vi "Moving_Statistic_Measurement.vi"(8 "error in (no error)":errorcluster, 10 "New_Measurement":dbl format="%#_13g", 11 "Moving_Mean in":refnum<class "Moving_Statistic.lvclass">) -> (0 "error out":errorcluster, 3 "Moving_Mean out":refnum<class "Moving_Statistic.lvclass">)   [LabVIEW 2021, in "Moving_Statistic.lvclass"]
uses:
  Moving_Statistic.lvclass
  Moving_Statistic.lvclass/Moving_Statistic.ctl
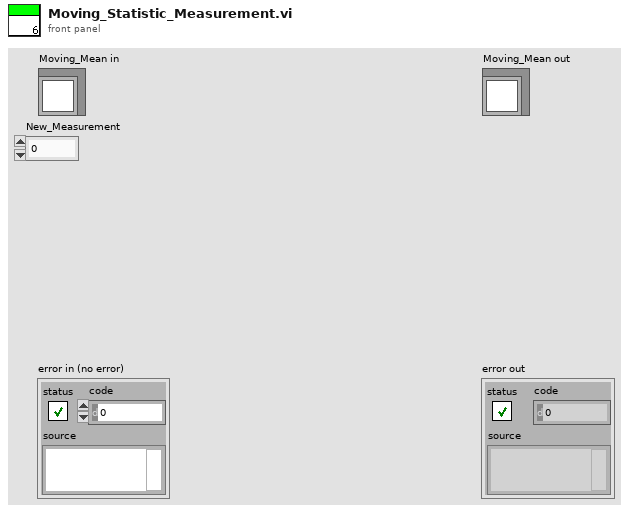
[diagram p1: front panel]
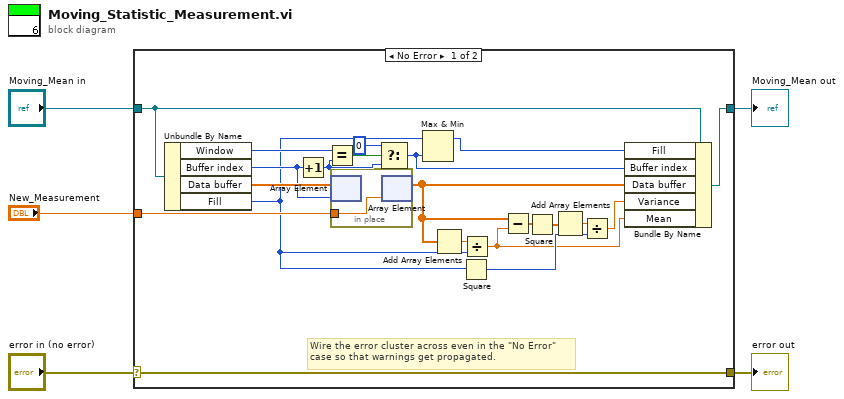
[diagram p0: block diagram]
diagram:
  n1 = case shown="No Error" "error in (no error)" {
    selector: "error in (no error)" -> [w26 w29]
    tunnel: [w26 w29] -> w4
    tunnel: [w10 w28] -> w2
    tunnel: "Moving_Mean in" -> [w9 w28]
    tunnel: "New_Measurement" -> [w25 _]
    frame No Error {
      # "Wire the error cluster across even in the \"No Error\"\ncase so that warnings get propagated."
      n2 = Unbundle By Name(w9) -> ("Window"=w23:i32, "Buffer index"=w22:i32, "Data buffer"=w24:dbl[], "Fill"=w15:i32)
      n3 = Increment(x=w22) -> (x+1=w19:i32)
      n4 = Equal?(x=w23, y=w19) -> (x = y?=w21:bool)
      n5 = in-place {
        in-place-border: w25 -> [w27]
        n6 = in-place-array #1(w24, w22) -> ()  [unwired: 1 out]
        n7 = in-place-array #1(w27) -> (w8:dbl[])  [unwired: 1 out]
      }
      n8 = Select(t=0, s=w21, f=w19) -> (s? t:f=w7:i32)
      n9 = Max & Min(x=w15, y=w7) -> (max(x,y)=w6:i32)  [unwired: 1 out]
      n10 = Add Array Elements(numeric array=w8) -> (sum=w18:dbl)
      n11 = Square(x=w15) -> (x^2=w13:i32)
      n12 = Divide(x=w18, y=w15) -> (x/y=w11:dbl)
      n13 = Subtract(x=w8, y=w11) -> (x-y=w17:dbl[])
      n14 = Square(x=w17) -> (x^2=w16:dbl[])
      n15 = Add Array Elements(numeric array=w16) -> (sum=w14:dbl)
      n16 = Divide(x=w14, y=w13) -> (x/y=w12:dbl)
      n17 = Bundle By Name(cluster=w9, "Fill"=w6, "Buffer index"=w7, "Data buffer"=w8, "Variance"=w12, "Mean"=w11) -> (w10:refnum<class "Moving_Statistic.lvclass">)
    }
    frame Error {
    }
  }
  "error out" <- w4
  "Moving_Mean out" <- w2
